vi "NestedCaseStructure.vi"   [LabVIEW 2017]
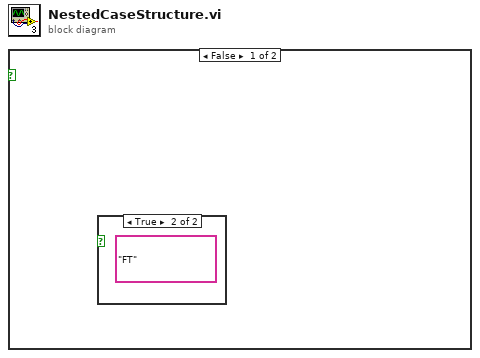
[diagram p0: block diagram]
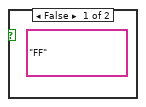
[diagram p2: hidden frame]
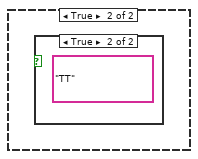
[diagram p3: hidden frame]
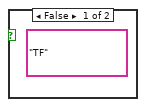
[diagram p4: hidden frame]
diagram:
  n1 = case shown="False" {
    selector: _ -> [_ _]
    frame False {
      n2 = case shown="True" {
        selector: _ -> [_ _]
        frame False {
          (unwired) "FF"
        }
        frame True {
          (unwired) "FT"
        }
      }
    }
    frame True {
      n3 = case shown="True" {
        selector: _ -> [_ _]
        frame False {
          (unwired) "TF"
        }
        frame True {
          (unwired) "TT"
        }
      }
    }
  }
